vi "Prompt User to Activate Web Server.vi"() -> (1 "Yes (T) / Cancel (F)":bool)   [LabVIEW 2026, in "Client Controller.lvlib" / "Client Controller.lvclass"]
uses:
  Client Controller.lvclass
  Client Controller.lvclass/Client Controller.ctl
panel:
  in  "Cancel Button":bool
  in  "OK Button":bool
  # "Since you appear to be running in the development environment,  please ensure you have started the web server."
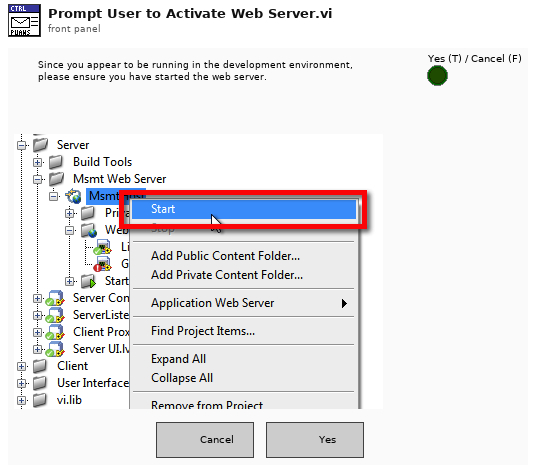
[diagram p1: front panel]
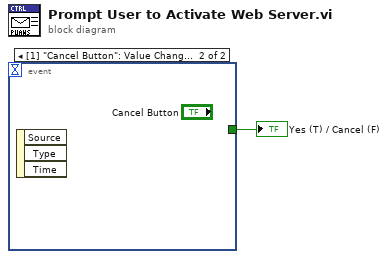
[diagram p0: block diagram]
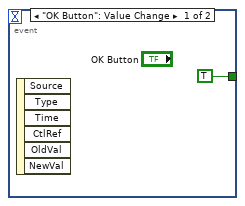
[diagram p2: hidden frame]
diagram:
  n1 = event shown="[1] \"Cancel Button\": Value Change;  Panel Close" {
    selector: _ -> [_ _]
    dyn-events: _ -> [_ _]
    timeout: _ -> [_ _]
    tunnel: [TRUE _] -> w1
    event "OK Button": Value Change {
      n2 = event-data() -> ()  [unwired: 1 in, 6 out]
    }
    event "Cancel Button": Value Change; Panel Close {
      n3 = event-data() -> ()  [unwired: 1 in, 3 out]
    }
  }
  "Yes (T) / Cancel (F)" <- w1
